vi "User Management CSV FGV.vi"(7 "Command":T2, 8 "error in (no error)":errorcluster, 9 "User data In":T1, 10 "Username":string, 11 "Path":path) -> (0 "error out":errorcluster, 1 "User data Out":T1, 2 "Usernames":string[](array[string]))   [LabVIEW 2017]
uses:
  Control/Login Authority CSV FGV Command.ctl
  <vilib>/Utility/file.llb/Write To Spreadsheet File (string).vi
  <vilib>/Utility/file.llb/Read From Spreadsheet File (string).vi
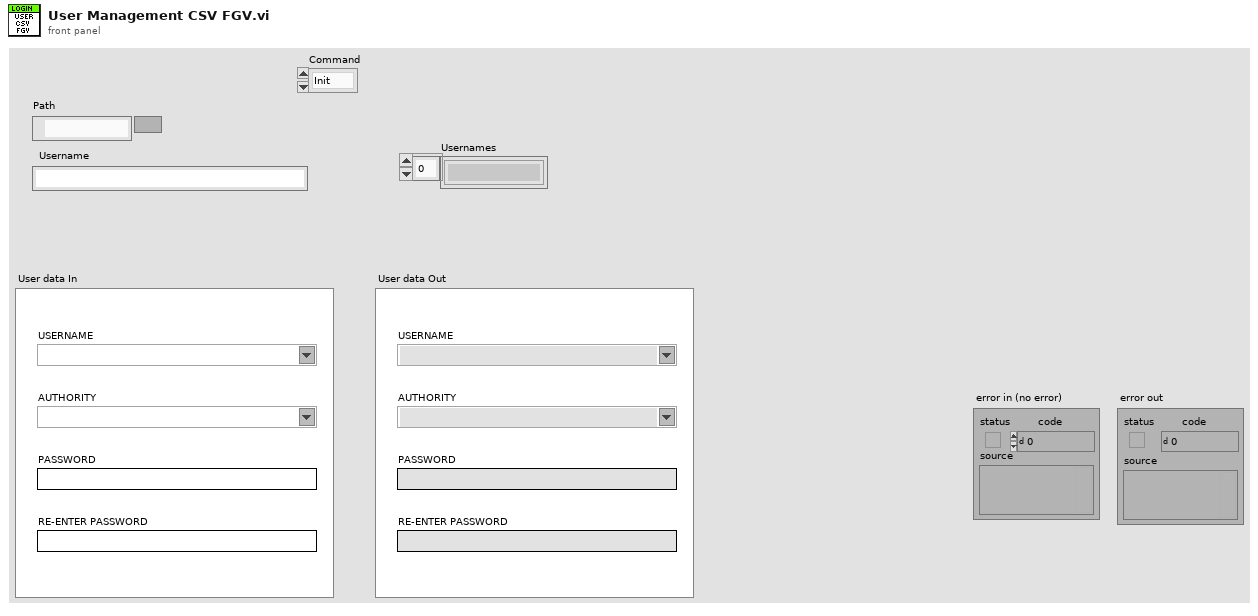
[diagram p1: front panel]
types:
  T1 = cluster{"USERNAME":string, "AUTHORITY":string, "PASSWORD":string, "RE-ENTER PASSWORD":string}
  T2 = typedef "Login Authority CSV FGV Command.ctl" = enum16{"Init", "Save", "Read", "Get Data", "Delete"}
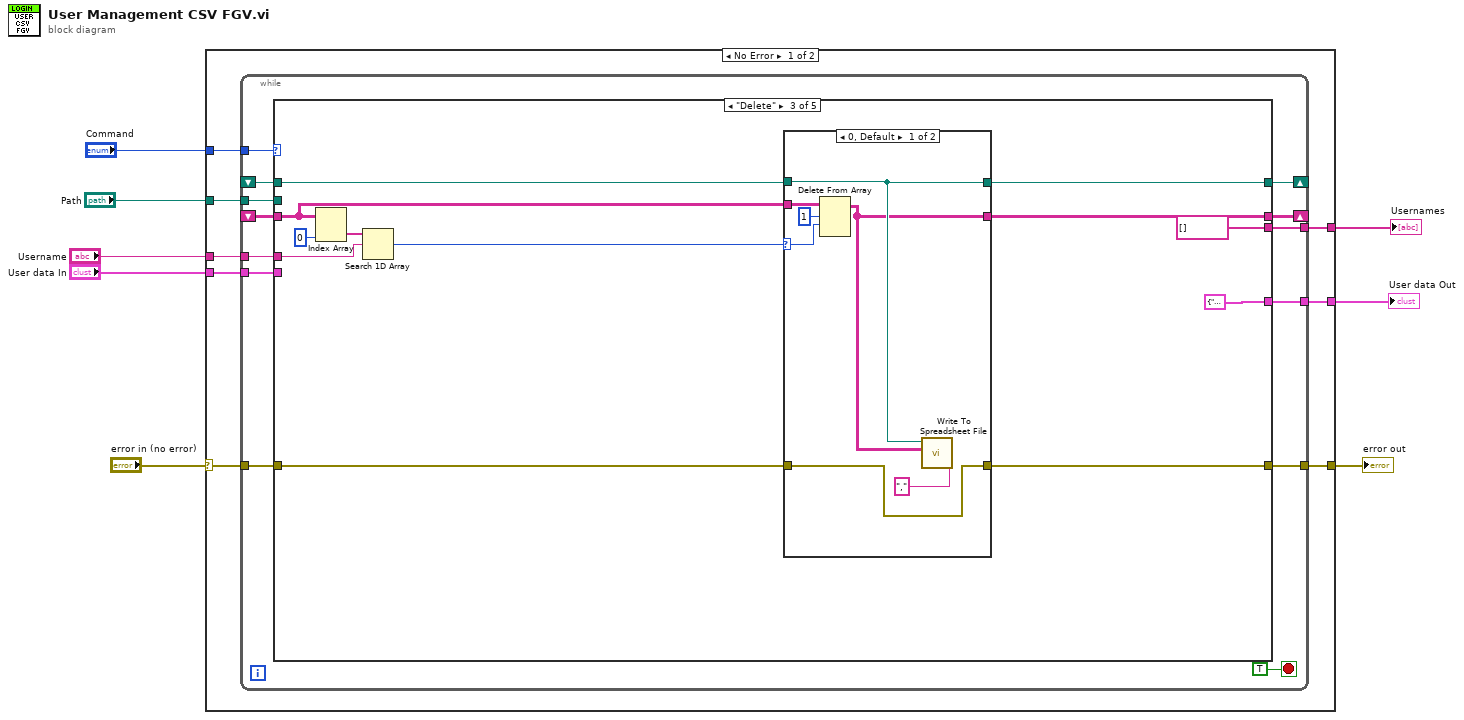
[diagram p0: block diagram]
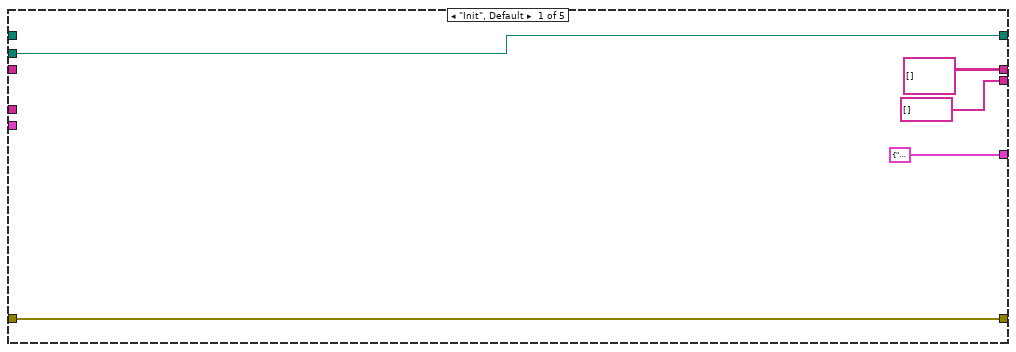
[diagram p2: hidden frame]
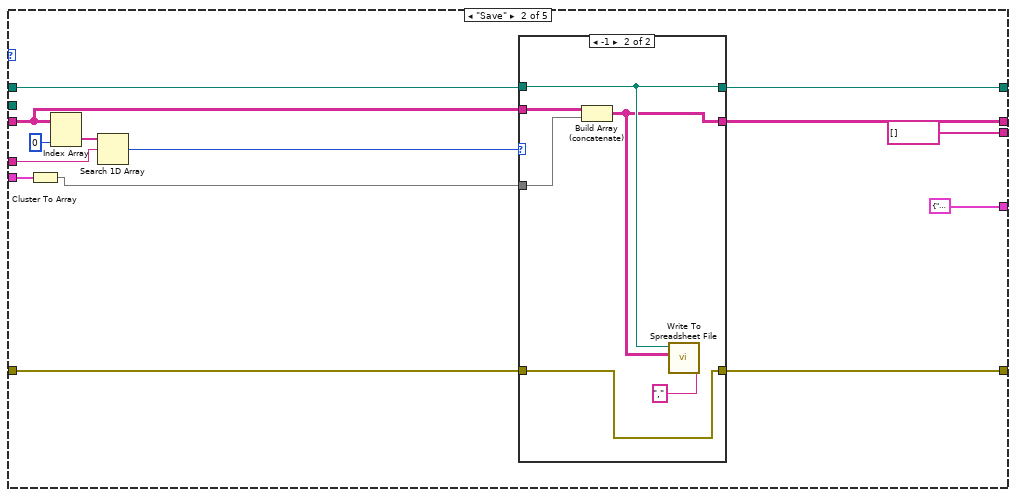
[diagram p3: hidden frame]
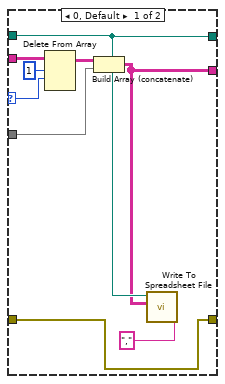
[diagram p4: hidden frame]
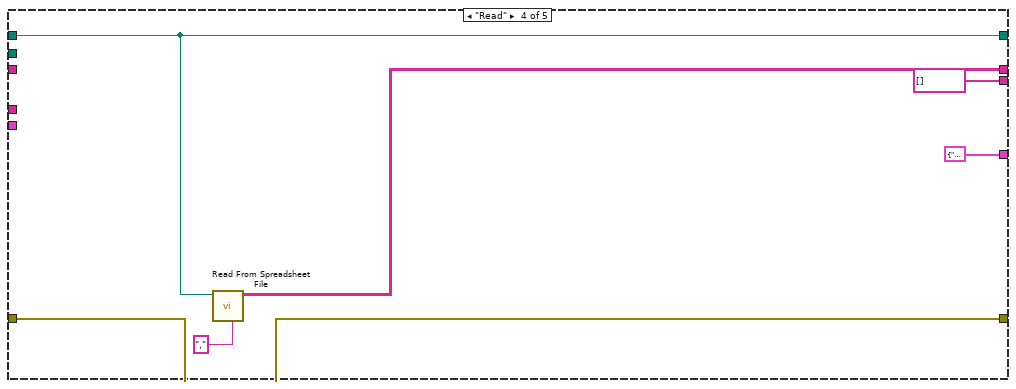
[diagram p6: hidden frame]
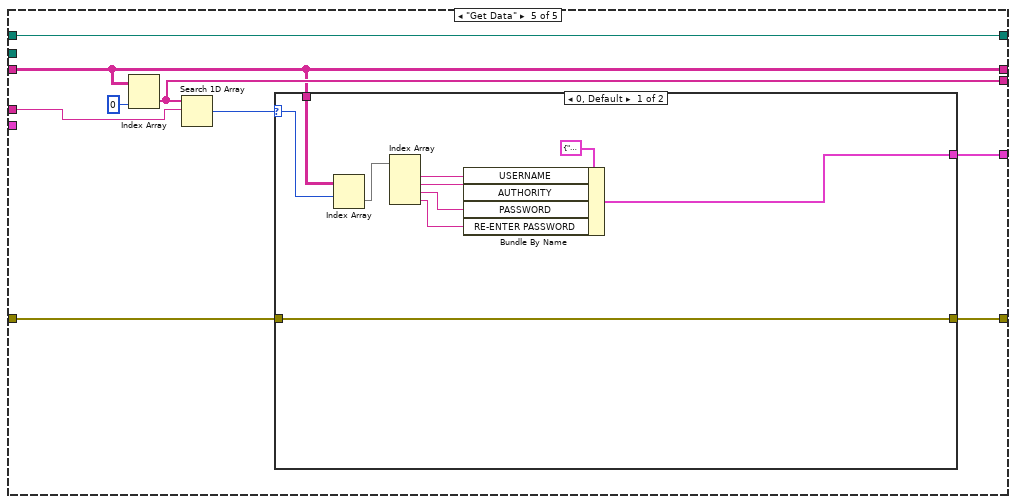
[diagram p7: hidden frame]
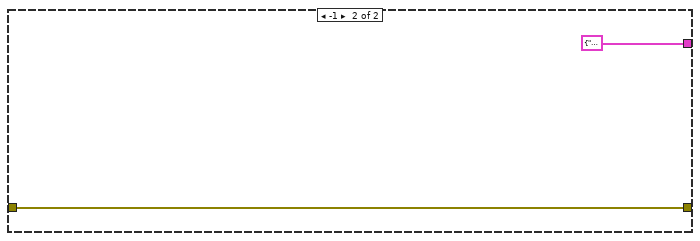
[diagram p8: hidden frame]
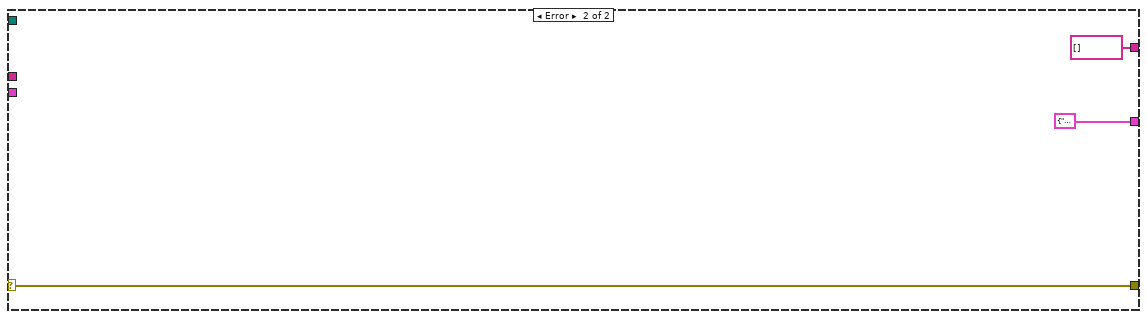
[diagram p9: hidden frame]
diagram:
  n1 = case shown="No Error" "error in (no error)" {
    selector: "error in (no error)" -> [w16 w115]
    tunnel: [w15 w115] -> w7
    tunnel: "Command" -> [w14 _]
    tunnel: "Path" -> [w10 _]
    tunnel: [w9 T1 {"USERNAME"="", "AUTHORITY"="", "PASSWORD"="", "RE-ENTER PASSWORD"=""} ("User data Out")] -> w1
    tunnel: "Username" -> [w13 _]
    tunnel: "User data In" -> [w12 _]
    tunnel: [w11 string[] [] ("all rows")] -> w3
    frame No Error {
      n2 = while {
        tunnel: w16 -> [w28]
        tunnel: [w27] -> w15
        tunnel: w14 -> [w26]
        shift-right: [w25] -> _
        shift-left: _ -> [w24]
        tunnel: w13 -> [w23]
        tunnel: w12 -> [w22]
        shift-right: [w18] -> _
        shift-left: _ -> [w21]
        tunnel: [w20] -> w11
        tunnel: w10 -> [w19]
        tunnel: [w17] -> w9
        stop <- TRUE stop-if-true
        n3 = case shown="\"Delete\"" w26 {
          tunnel: w28 -> [w34 w39 w71 w87 w96]
          tunnel: [w34 w44 w68 w87 w95] -> w27
          tunnel: [w33 w42 w69 w90 w100] -> w25
          tunnel: w24 -> [_ w43 w70 w90 w100]
          tunnel: w23 -> [_ w37 w73 _ w98]
          tunnel: w22 -> [_ w38 _ _ _]
          tunnel: [string[][] [] w45 w66 w86 w93] -> w18
          tunnel: w21 -> [_ w46 w72 _ w93]
          tunnel: [string[] [] ("all rows") string[] [] ("all rows") string[] [] ("all rows") string[] [] ("all rows") w97] -> w20
          tunnel: w19 -> [w33 _ _ _ _]
          tunnel: [T1 {"USERNAME"="", "AUTHORITY"="", "PASSWORD"="", "RE-ENTER PASSWORD"=""} ("User data Out") T1 {"USERNAME"="", "AUTHORITY"="", "PASSWORD"="", "RE-ENTER PASSWORD"=""} ("User data Out") T1 {"USERNAME"="", "AUTHORITY"="", "PASSWORD"="", "RE-ENTER PASSWORD"=""} ("User data Out") T1 {"USERNAME"="", "AUTHORITY"="", "PASSWORD"="", "RE-ENTER PASSWORD"=""} ("User data Out") w92] -> w17
          frame "Init", Default {
          }
          frame "Save" {
            n4 = Cluster To Array(cluster=w38) -> (array=w35:string[])
            n5 = Index Array(array=w46, index (col)=0 ("disabled index (col)")) -> (element=w41:string[])  [unwired: 1 in]
            n6 = Search 1D Array(1D array=w41, element=w37) -> (index of element=w47:i32)  [unwired: 1 in]
            n7 = case shown="-1" w47 {
              selector: w47 -> [w53 _]
              tunnel: w46 -> [w57 w63]
              tunnel: [w49 w58] -> w45
              tunnel: [w50 w59] -> w44
              tunnel: w43 -> [w54 w61]
              tunnel: [w54 w61] -> w42
              tunnel: w35 -> [w51 w60]
              tunnel: w39 -> [w50 w59]
              frame 0, Default {
                n8 = Delete From Array(array=w57, length=1, index (row)=w53) -> (array with subset deleted=w56:string[][])  [unwired: 1 in, 1 out]
                n9 = Build Array (concatenate)(w56, w51) -> (w49:string[][])
                n10 = call-poly <vilib>:"Write To Spreadsheet File.vi"("delimiter (\\t)"="," ("delimiter (\\t)"), "2D data"=w49, "file path (dialog if empty)"=w54) -> ()  [unwired: 5 in, 1 out]
              }
              frame -1 {
                n11 = Build Array (concatenate)(w63, w60) -> (w58:string[][])
                n12 = call-poly <vilib>:"Write To Spreadsheet File.vi"("delimiter (\\t)"="," ("delimiter (\\t)"), "2D data"=w58, "file path (dialog if empty)"=w61) -> ()  [unwired: 5 in, 1 out]
              }
            }
          }
          frame "Delete" {
            n13 = Index Array(array=w72, index (col)=0 ("disabled index (col)")) -> (element=w65:string[])  [unwired: 1 in]
            n14 = Search 1D Array(1D array=w65, element=w73) -> (index of element=w74:i32)  [unwired: 1 in]
            n15 = case shown="0, Default" w74 {
              selector: w74 -> [w78 _]
              tunnel: w72 -> [w82 w84]
              tunnel: [w76 w84] -> w66
              tunnel: w71 -> [w77 w83]
              tunnel: w70 -> [w80 w85]
              tunnel: [w80 w85] -> w69
              tunnel: [w77 w83] -> w68
              frame 0, Default {
                n16 = Delete From Array(array=w82, length=1, index (row)=w78) -> (array with subset deleted=w76:string[][])  [unwired: 1 in, 1 out]
                n17 = call-poly <vilib>:"Write To Spreadsheet File.vi"("delimiter (\\t)"="," ("delimiter (\\t)"), "2D data"=w76, "file path (dialog if empty)"=w80) -> ()  [unwired: 5 in, 1 out]
              }
              frame -1 {
              }
            }
          }
          frame "Read" {
            n18 = call-poly <vilib>:"Read From Spreadsheet File.vi"("delimiter (\\t)"="," ("delimiter (\\t)"), "file path (dialog if empty)"=w90) -> ("all rows"=w86:string[][])  [unwired: 5 in, 4 out]
          }
          frame "Get Data" {
            n19 = Index Array(array=w93, index (col)=0 ("disabled index (col)")) -> (element=w97:string[])  [unwired: 1 in]
            n20 = Search 1D Array(1D array=w97, element=w98) -> (index of element=w94:i32)  [unwired: 1 in]
            n21 = case shown="0, Default" w94 {
              selector: w94 -> [w109 _]
              tunnel: w96 -> [w108 w112]
              tunnel: [w108 w112] -> w95
              tunnel: w93 -> [w110 _]
              tunnel: [w101 T1 {"USERNAME"="", "AUTHORITY"="", "PASSWORD"="", "RE-ENTER PASSWORD"=""} ("User data Out")] -> w92
              frame 0, Default {
                n22 = Index Array(array=w110, index (row)=w109) -> (element=w106:string[])  [unwired: 1 in]
                n23 = Index Array(array=w106) -> (element #1=w105:string, element #2=w104:string, element #3=w103:string, element #4=w102:string)  [unwired: 4 in]
                n24 = Bundle By Name(cluster=T1 {"USERNAME"="", "AUTHORITY"="", "PASSWORD"="", "RE-ENTER PASSWORD"=""} ("User data Out"), "USERNAME"=w105, "AUTHORITY"=w104, "PASSWORD"=w103, "RE-ENTER PASSWORD"=w102) -> (w101:T1)
              }
              frame -1 {
              }
            }
          }
        }
      }
    }
    frame Error {
    }
  }
  "error out" <- w7
  "Usernames" <- w3
  "User data Out" <- w1
